vi "Read LS 325.vi"() -> ()   [LabVIEW 2017]
uses:
  <instrlib>/Lake Shore 325/Lake Shore 325.lvlib
  <instrlib>/Lake Shore Cryotronics 331/Lake Shore Cryotronics 331.lvlib
panel:
  in  "?":u16(ring) items=["Kelvin", "Celsius", "Sensor Units"]
  in  "Sensor Input (0:A)":u16(ring) items=["A", "B"]
  out "error out":errorcluster
  in  "error in (no error)":errorcluster
  out "Sensor Data":dbl format="%.4f"
  in  "Serial Configuration":T1={"Baud Rate"=9600, "Parity"=1, "Data Bits"=7, "Stop Bits"=10, "Flow Control"=0} {"Flow Control" items=["None", "XON/XOFF", "RTS/CTS", "XON/XOFF & RTS/CTS", "DTR/DSR", "XON/XOFF & DTR/DSR"]; "Stop Bits" items=["1.0"=10, "1.5"=15, "2.0"=20]; "Data Bits" items=["7"=7, "8"=8]; "Parity" items=["None", "Odd", "Even", "Mark", "Space"]; "Baud Rate" items=["300"=300, "600"=600, "1200"=1200, "2400"=2400, "4800"=4800, "9600"=9600, "19200"=19200, "38400"=38400, "57600"=57600]}
  in  "325 VISA resource":refnum<visa-resource-name>="COM3"
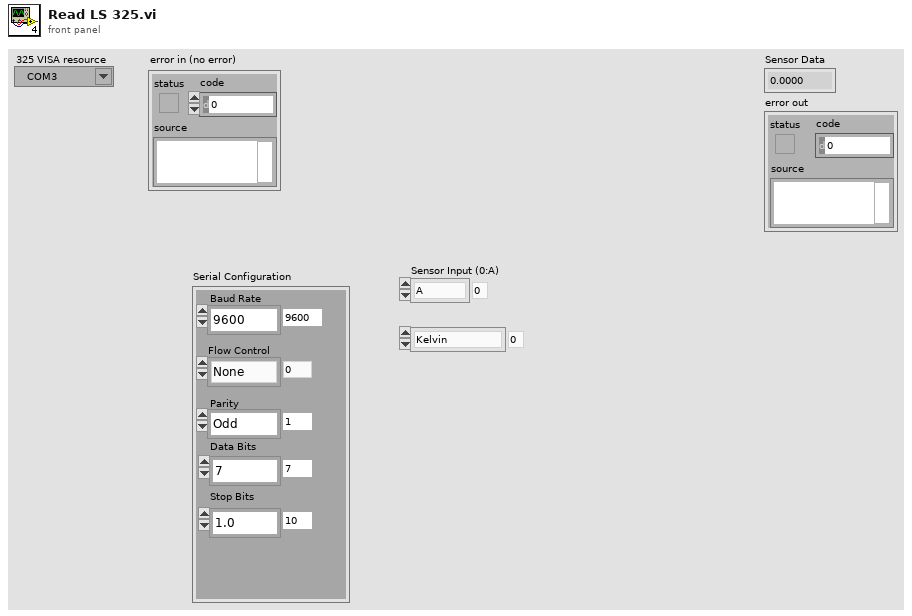
[diagram p1: front panel]
types:
  T1 = cluster{"Baud Rate":u32, "Parity":u16, "Data Bits":u16, "Stop Bits":u16, "Flow Control":u16}
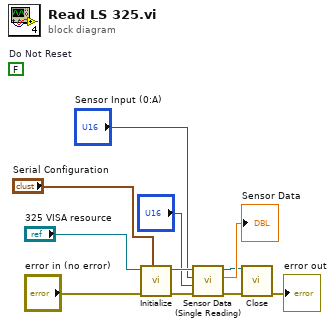
[diagram p0: block diagram]
diagram:
  (unwired) FALSE  # Do Not Reset
  n1 = call <instrlib>:"Initialize.vi"("Serial Configuration"="Serial Configuration", "error in (no error)"="error in (no error)", "VISA resource name"="325 VISA resource") -> ("error out"=w7:errorcluster, "VISA resource name out"=w10:refnum<visa-resource-name>)  [unwired: 7 in]
  n2 = call <instrlib>:"Sensor Data (Single Reading).vi"("error in (no error)"=w7, "Data Source (0:Kelvin)"="?", "Sensor Input (0:A)"="Sensor Input (0:A)", "VISA resource name"=w10) -> ("error out"=w3:errorcluster, "Sensor Data"=→"Sensor Data":dbl, "VISA resource name out"=w2:refnum<visa-resource-name>)  [unwired: 5 in]
  n3 = call <instrlib>:"Close.vi"("VISA resource name"=w2, "error in (no error)"=w3) -> ("error out"=→"error out":errorcluster)  [unwired: 13 in]
